vi "Write RepoName.vi"(8 "error in (no error)":errorcluster, 10 "RepoName":string, 11 "Package Version in":refnum<class "Package Version.lvclass">) -> (0 "error out":errorcluster, 3 "Package Version out":refnum<class "Package Version.lvclass">)   [LabVIEW 2020, in "Packages.lvlib" / "Package Version.lvclass"]
uses:
  Package Version.lvclass
  Package Version.lvclass/Package Version.ctl
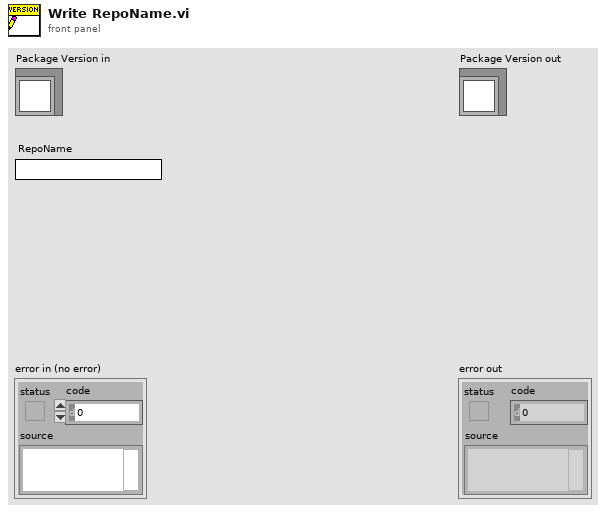
[diagram p1: front panel]
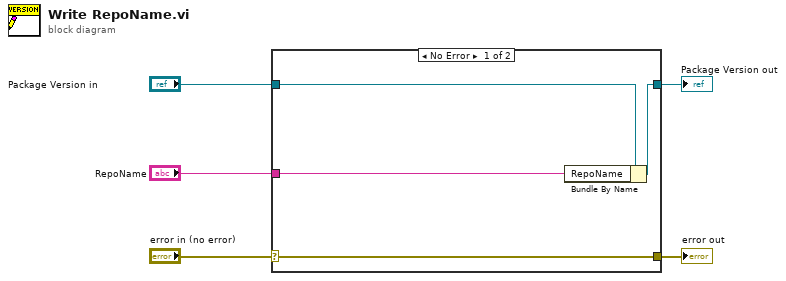
[diagram p0: block diagram]
diagram:
  n1 = case shown="No Error" "error in (no error)" {
    selector: "error in (no error)" -> [w9 w10]
    tunnel: [w9 w10] -> w4
    tunnel: [w7 w11] -> w2
    tunnel: "Package Version in" -> [w8 w11]
    tunnel: "RepoName" -> [w6 _]
    frame No Error {
      n2 = Bundle By Name(cluster=w8, "RepoName"=w6) -> (w7:refnum<class "Package Version.lvclass">)
    }
    frame Error {
    }
  }
  "error out" <- w4
  "Package Version out" <- w2
